vi "Launcher.vi"() -> ()   [LabVIEW 2021, in "Echo Broadcast Test Without Server Manager.lvlib"]
uses:
  Echo Broadcast Test Without Server Manager.lvlib
  WebSocket Actor/WebSocket Server/WebSocket Server.lvclass
  C:/Program Files/National Instruments/LabVIEW 2021/vi.lib/ActorFramework/Actor/Actor.lvclass
  WS Test Server/WS Test Server.lvclass
  WS Test Server Messages/Server Connection Handler Msg/Server Connection Handler Msg.lvclass
  C:/Projects/WebSocket-Actor/WebSocket Actor/Abstract Messages/WebSocket Connection Handler Msg/WebSocket Connection Handler Msg.lvclass
  WebSocket Actor/WebSocket Server/typedefs/Listener Settings.ctl
  WebSocket Actor/WebSocket Server/WebSocket Server.lvclass/WebSocket Server.ctl
  WS Test Client/WS Test Client.lvclass
  WebSocket Actor/WebSocket Client/WebSocket Client.lvclass
  C:/Projects/WebSocket-Actor/WebSocket Actor/WebSocket Connection/WebSocket Connection.lvclass
  WS Test Client Messages/Client Connection Handler Msg/Client Connection Handler Msg.lvclass
  WebSocket Actor/WebSocket Connection/WebSocket Connection.lvclass/WebSocket Connection.ctl
  <vilib>/ActorFramework/Message Enqueuer/Message Enqueuer.lvclass/Message Enqueuer.ctl
  WebSocket Actor/WebSocket Connection/properties/Write Timeout.vi
  WebSocket Actor/WebSocket Connection/properties/Write WebSocket Data Handler.vi
  WebSocket Actor/WebSocket Server/properties/Write Listener Settings.vi
  WebSocket Actor/WebSocket Server/properties/Write Handshake timeout (5000 ms).vi
  <vilib>/ActorFramework/Message Enqueuer/Enqueue.vi
  <vilib>/ActorFramework/Stop Msg/Stop Msg.lvclass
  C:/Program Files/National Instruments/LabVIEW 2021/vi.lib/ActorFramework/Message/Message.lvclass
  WebSocket Actor/WebSocket Client/properties/Write WS URI.vi
  <vilib>/Utility/LVClass/Get LV Class Name.vi
  <resource>/AFDebug/Generate Trace for Message.vi
  <vilib>/ActorFramework/Message Priority Queue/Priority Enqueue.vi
  <vilib>/ActorFramework/Actor/Actor.lvclass
  WebSocket Actor/WebSocket Server Messages/Add Service Msg/Add Service Msg.lvclass
  <userlib>/_OpenG.lib/time/time.llb/openg_time.lvlib
  C:/Projects/WebSocket-Actor/Examples/Echo Broadcast Test Without Server Manager/WS Test Server/WS Test Server.lvclass
  C:/Projects/WebSocket-Actor/WebSocket Actor/WebSocket Server/WebSocket Server.lvclass
  C:/Projects/WebSocket-Actor/Examples/Echo Broadcast Test Without Server Manager/WS Test Server Messages/Server Connection Handler Msg/Server Connection Handler Msg.lvclass
  C:/Projects/WebSocket-Actor/Examples/Echo Broadcast Test Without Server Manager/WS Test Client/WS Test Client.lvclass
  C:/Projects/WebSocket-Actor/Examples/Echo Broadcast Test Without Server Manager/WS Test Client Messages/Client Connection Handler Msg/Client Connection Handler Msg.lvclass
  C:/Projects/WebSocket-Actor/WebSocket Actor/WebSocket Client/WebSocket Client.lvclass
  WebSocket Actor/WebSocket Connection/Keepalive.ctl
  WebSocket Actor/WebSocket Connection/WebSocket Connection.lvclass
panel:
  in  "Keepalive":T1={"Enabled"=TRUE, "Ping Interval (ms)"=25000, "Ping Timeout (ms)"=20000}
  in  "Stop Server":bool
  in  "Number of Clients":i32=3
  # "In this example we will  launch WebSocket server (without the Server Manager Actor Infrastructure) and we will illustrate a bidirectional communication between WebSocket server and clients. \nWe launch one server that will define the /echo/ service. Then a user selectable number of client can be launched. From such clients messages to the servers can be sent on the specified service. The server will echo back the message to the clients. \nInstructions to execute the example:\n\n1. Run this VI\n2. Wait that the Client's GUI appear\n3. use the GUIs to exchange messages\n4. Stop running Actors form this VI"
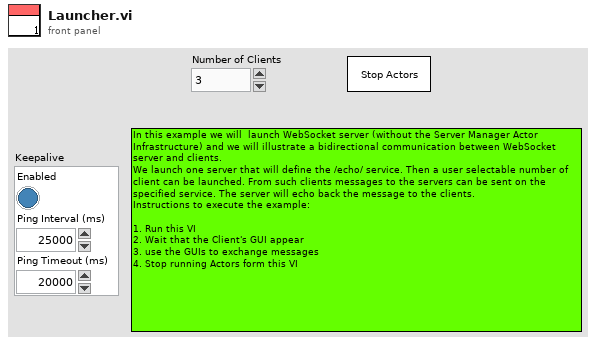
[diagram p1: front panel]
types:
  T1 = typedef "WebSocket Actors.lvlib/WebSocket Connection.lvclass/Keepalive.ctl" = cluster{"Enabled":bool, "Ping Interval (ms)":u32, "Ping Timeout (ms)":u32}
  T2 = typedef "WebSocket Actors.lvlib/WebSocket Server.lvclass/Listener Settings.ctl" = cluster{"resolve remote address (T)":bool, "timeout ms (-1)":i32, "net address":u32, "port":u16}
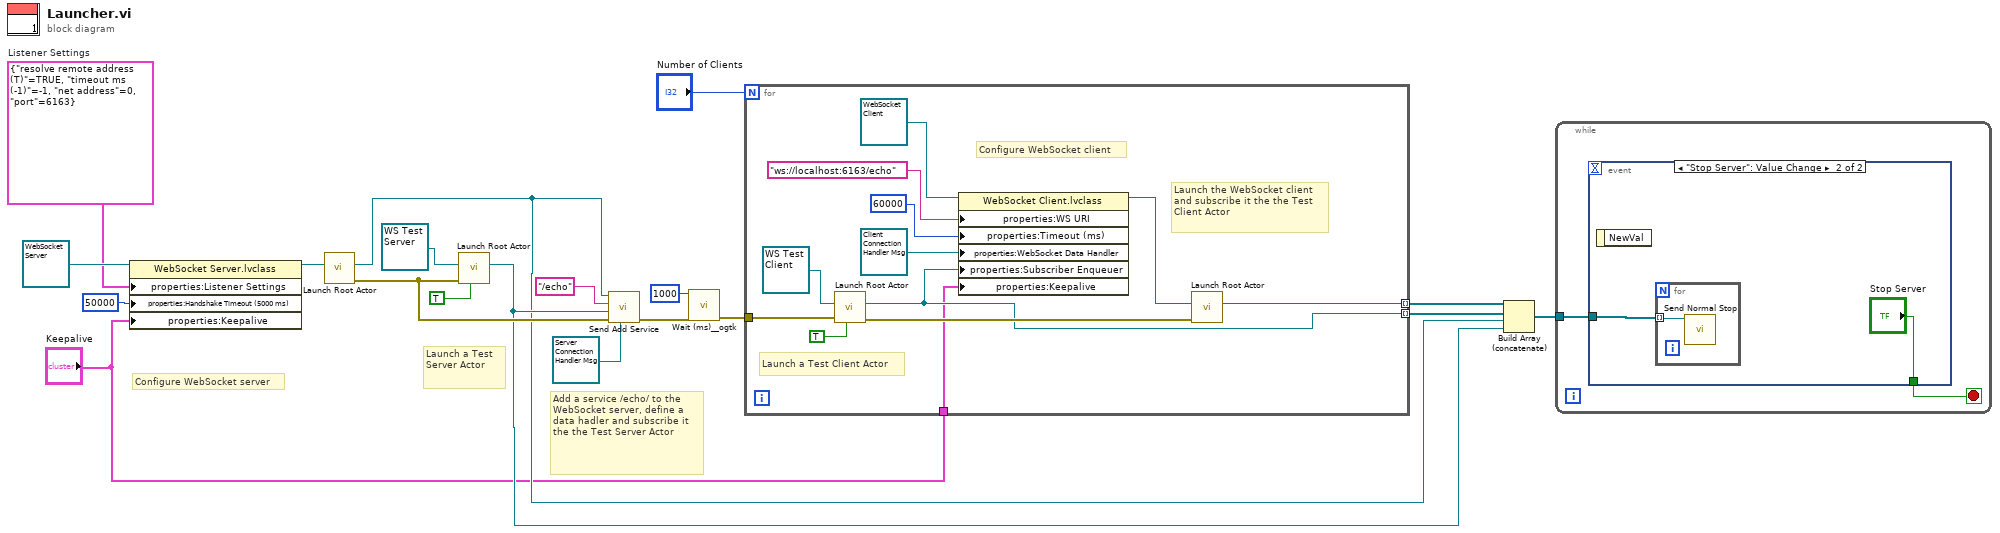
[diagram p0: block diagram]
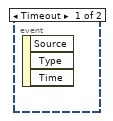
[diagram p2: hidden frame]
diagram:
  w12 = T2 {"resolve remote address (T)"=TRUE, "timeout ms (-1)"=-1, "net address"=0, "port"=6163}  # Listener Settings
  # "Launch a Test Server Actor"
  # "Add a service /echo/ to the WebSocket server, define a data hadler and subscribe it the the Test Server Actor"
  # "Configure WebSocket server"
  n1 = property class="WebSocket Server.lvclass"(reference=refnum<class "WebSocket Server.lvclass"> refnum ("WebSocket Actors.lvlib:WebSocket Server.lvclass"), "properties:Listener Settings"=w12, "properties:Handshake Timeout (5000 ms)"=50000 ("Handshake timeout (5000 ms)"), "properties:Keepalive"="Keepalive") -> (reference out=w13:refnum<class "WebSocket Server.lvclass">)  [unwired: 1 in, 1 out]
  n2 = call <vilib>:"Launch Root Actor.vi"("Actor"=w13) -> ("error out"=w16:errorcluster, "Actor's Enqueuer"=w4:refnum<class "Message Enqueuer.lvclass">)  [unwired: 9 in]
  n3 = call <vilib>:"Launch Root Actor.vi"("Open Actor Core front panel? (F)"=TRUE, "error in (no error)"=w16, "Actor"=refnum<class "WS Test Server.lvclass"> refnum ("WS Full LabVIEW Test.lvlib:WS Test Server.lvclass")) -> ("Actor's Enqueuer"=w5:refnum<class "Message Enqueuer.lvclass">)  [unwired: 7 in, 1 out]
  n4 = call "Send Add Service.vi"("WebSocket Data Handler"=refnum<class "Server Connection Handler Msg.lvclass"> refnum ("WS Full LabVIEW Test.lvlib:Server Connection Handler Msg.lvclass"), "error in (no error)"=w16, "Subscriber Enqueuer"=w5, "Service Name"="/echo", "Message Enqueuer in"=w4) -> ("error out"=w8:errorcluster)  [unwired: 5 in, 1 out]
  n5 = call <userlib>:"Wait (ms)__ogtk.vi"("error in (no error)"=w8, "milliseconds to wait"=u32 1000) -> ("error out"=w7:errorcluster)  [unwired: 8 in, 1 out]
  n6 = for {
    N: "Number of Clients" -> [_]
    tunnel: w7 -> [w24]
    tunnel: [w22] -> w6 mode=indexing
    tunnel: [w21] -> w2 mode=indexing
    tunnel: "Keepalive" -> [w20]
    # "Launch the WebSocket client and subscribe it the the Test Client Actor"
    # "Configure WebSocket client"
    # "Launch a Test Client Actor"
    n7 = call <vilib>:"Launch Root Actor.vi"("Open Actor Core front panel? (F)"=TRUE, "error in (no error)"=w24, "Actor"=refnum<class "WS Test Client.lvclass"> refnum ("WS Full LabVIEW Test.lvlib:WS Test Client.lvclass")) -> ("error out"=w25:errorcluster, "Actor's Enqueuer"=w21:refnum<class "Message Enqueuer.lvclass">)  [unwired: 7 in]
    n8 = property class="WebSocket Client.lvclass"(reference=refnum<class "WebSocket Client.lvclass"> refnum ("WebSocket Actors.lvlib:WebSocket Client.lvclass"), "properties:WS URI"="ws://localhost:6163/echo" ("Address"), "properties:Timeout (ms)"=60000 ("Timeout (60000 ms)"), "properties:WebSocket Data Handler"=refnum<class "Client Connection Handler Msg.lvclass"> refnum ("WS Full LabVIEW Test.lvlib:Client Connection Handler Msg.lvclass"), "properties:Subscriber Enqueuer"=w21, "properties:Keepalive"=w20) -> (reference out=w27:refnum<class "WebSocket Client.lvclass">)  [unwired: 1 in, 1 out]
    n9 = call <vilib>:"Launch Root Actor.vi"("error in (no error)"=w25, "Actor"=w27) -> ("Actor's Enqueuer"=w22:refnum<class "Message Enqueuer.lvclass">)  [unwired: 8 in, 1 out]
  }
  n10 = Build Array (concatenate)(w6, w2, w4, w5) -> (w3:refnum<class "Message Enqueuer.lvclass">[])
  n11 = while {
    tunnel: w3 -> [w33]
    stop <- w32 stop-if-true
    n12 = event shown="[1] \"Stop Server\": Value Change" {
      selector: _ -> [_ _]
      dyn-events: _ -> [_ _]
      timeout: _ -> [_ _]
      tunnel: w33 -> [_ w35]
      tunnel: [_ "Stop Server"] -> w32
      event Timeout {
        n13 = event-data() -> ()  [unwired: 1 in, 3 out]
      }
      event "Stop Server": Value Change {
        n14 = event-data() -> ()  [unwired: 1 in, 1 out]
        n15 = for {
          tunnel: w35 -> [w36] mode=indexing
          n16 = call <vilib>:"Send Normal Stop.vi"("Message Enqueuer"=w36) -> ()  [unwired: 10 in, 1 out]
        }
      }
    }
  }
